vi "GoToAngle.vi"(10 "Target Angle":dbl, 11 "Current Angle":dbl) -> ()   [LabVIEW 2016]
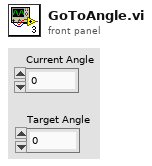
[diagram p1: front panel]
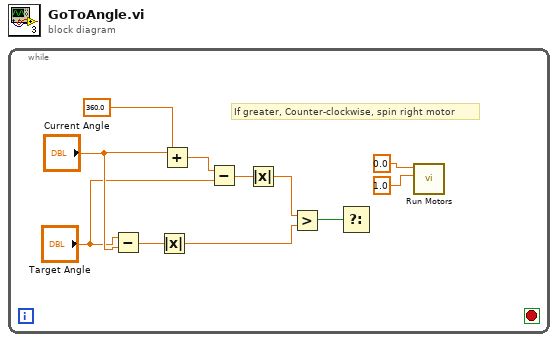
[diagram p0: block diagram]
diagram:
  n1 = while {
    stop <- _ stop-if-true
    # "If greater, Counter-clockwise, spin right motor"
    n2 = Subtract(x="Target Angle", y="Current Angle") -> (x-y=w7:dbl)
    n3 = Absolute Value(x=w7) -> (abs(x)=w2:dbl)
    n4 = Add(x="Current Angle", y=360.0) -> (x+y=w6:dbl)
    n5 = Subtract(x=w6, y="Target Angle") -> (x-y=w4:dbl)
    n6 = Absolute Value(x=w4) -> (abs(x)=w3:dbl)
    n7 = Greater?(x=w3, y=w2) -> (0:w1:bool)
    n8 = Select(s=w1) -> ()  [unwired: 2 in, 1 out]
    n9 = call "Run Motors.vi"("Right motor side (-1..1)"=1.0, "Left motor speed (-1..1)"=0.0) -> ()  [unwired: 10 in]
  }
